vi "RunHTOutconter.vi"() -> ()   [LabVIEW 2012]
uses:
  <vilib>/Utility/file.llb/Read From Spreadsheet File (string).vi
  <vilib>/regexp/Match Regular Expression.xnode
panel:
  out "concatenated string 4":string
  out "filenames":string[](array[string])
  out "concatenated string 3":string
  out "concatenated string 2":string
  out "concatenated string":string
  in  "file path (dialog if empty)":path=path "C:/temp/ht/now/HTentity.txt"
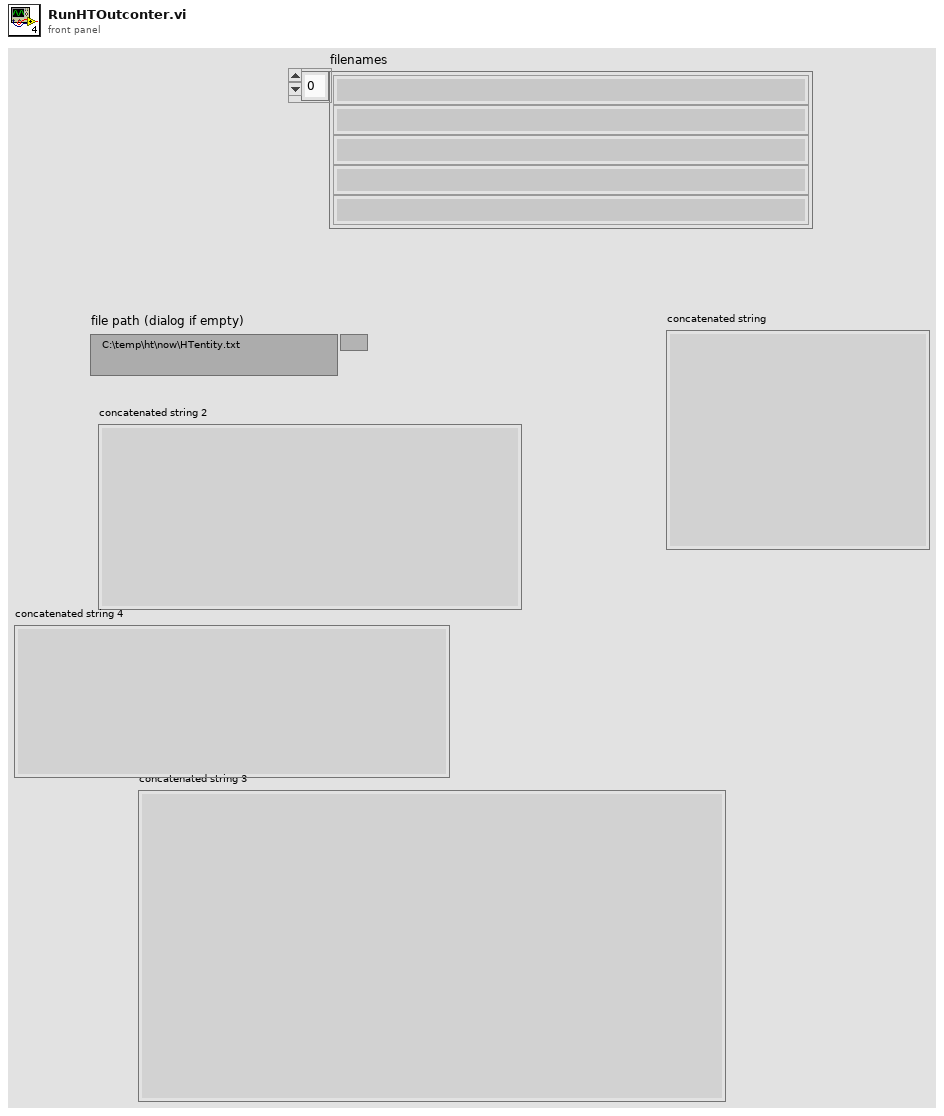
[diagram p1: front panel]
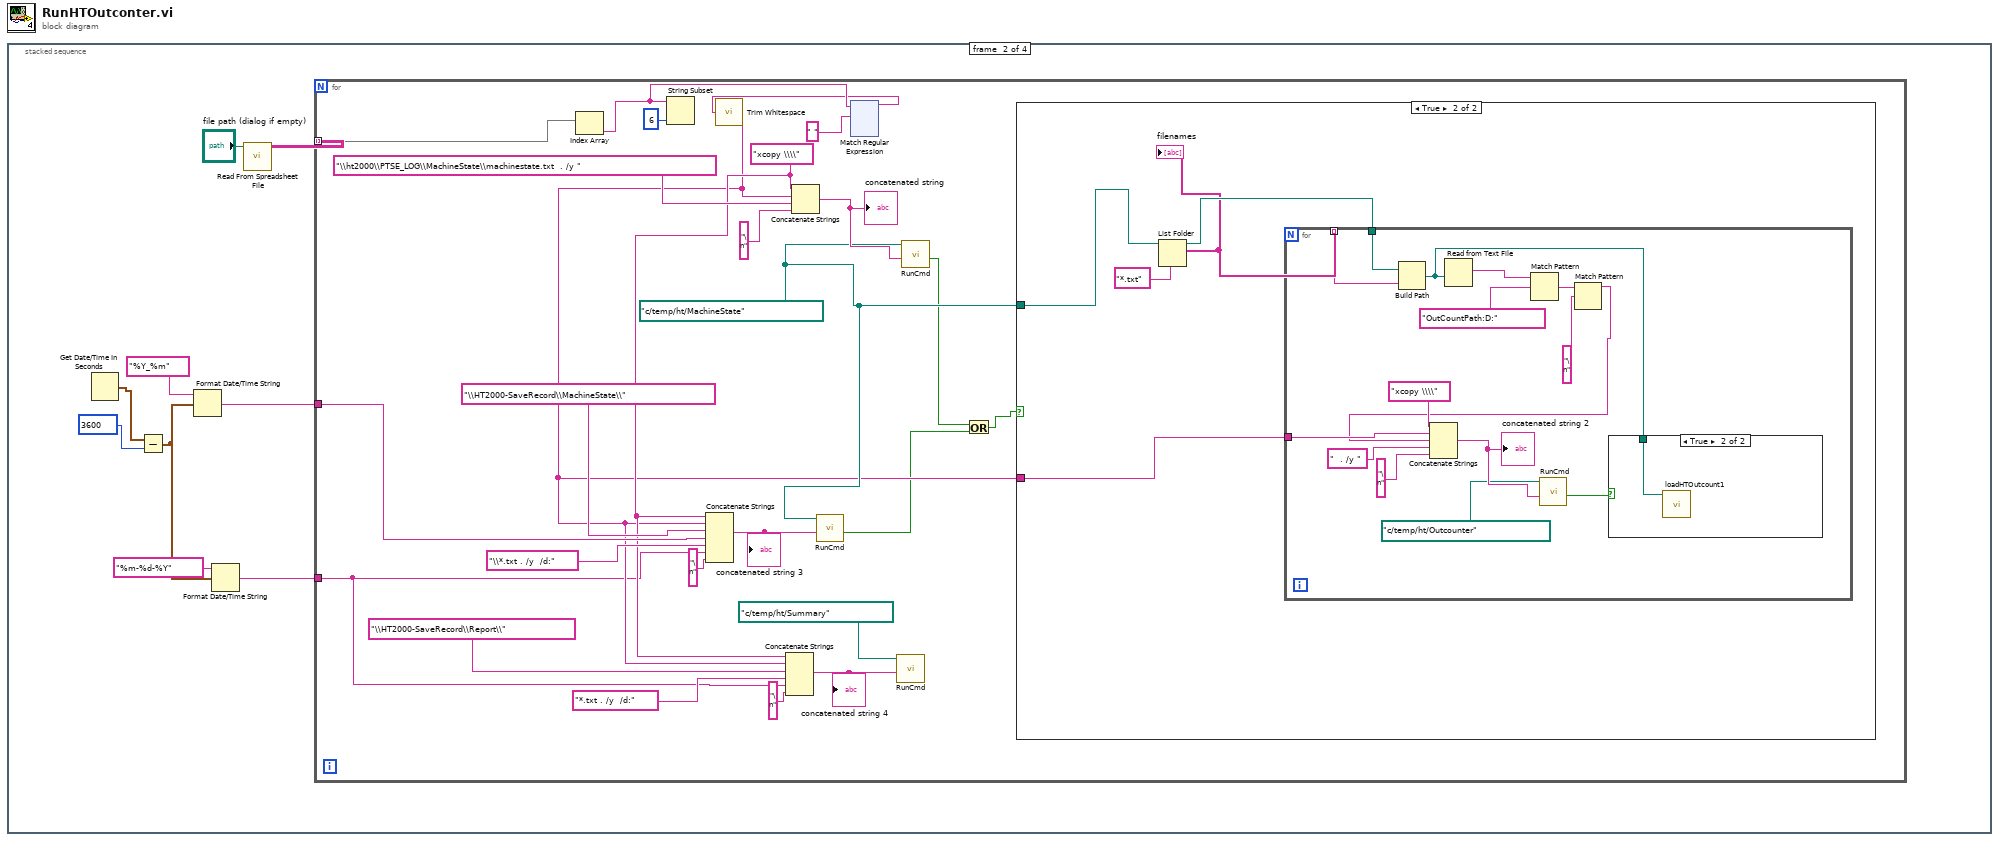
[diagram p0: block diagram]
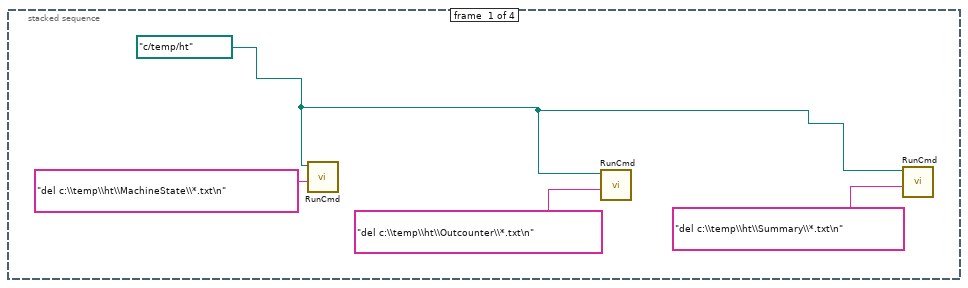
[diagram p2: hidden frame]
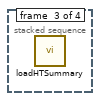
[diagram p5: hidden frame]
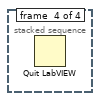
[diagram p6: hidden frame]
diagram:
  n1 = stacked-sequence {
    frame #0 {
      w1 = path "c:/temp/ht" ("working directory")
      n2 = call "RunCmd.vi"("Cmd String"="del c:\\temp\\ht\\MachineState\\*.txt\n", "working directory"=w1) -> ()  [unwired: 8 in, 2 out]
      n3 = call "RunCmd.vi"("Cmd String"="del c:\\temp\\ht\\Outcounter\\*.txt\n", "working directory"=w1) -> ()  [unwired: 8 in, 2 out]
      n4 = call "RunCmd.vi"("Cmd String"="del c:\\temp\\ht\\Summary\\*.txt\n", "working directory"=w1) -> ()  [unwired: 8 in, 2 out]
    }
    frame #1 {
      n5 = Get Date/Time In Seconds() -> (seconds since 1Jan1904=w10:timestamp)
      n6 = Subtract(x=w10, y=3600) -> (x-y=w7:timestamp)
      n7 = Format Date/Time String(time format string (%c)="%Y_%m", seconds (now)=w7) -> (date/time string=w8:string)  [unwired: 1 in]
      n8 = Format Date/Time String(time format string (%c)="%m-%d-%Y", seconds (now)=w7) -> (date/time string=w5:string)  [unwired: 1 in]
      n9 = call-poly <vilib>:"Read From Spreadsheet File.vi"("file path (dialog if empty)"="file path (dialog if empty)") -> ("all rows"=w13:string[][])  [unwired: 6 in, 4 out]
      n10 = for {
        tunnel: w13 -> [w35] mode=indexing
        tunnel: w8 -> [w29]
        tunnel: w5 -> [w19]
        w27 = path "c:/temp/ht/MachineState" ("working directory")
        w23 = "xcopy \\\\" ("string")
        n11 = Index Array(array=w35) -> (element=w33:string)  [unwired: 1 in]
        n12 = String Subset(string=w33, length (rest)=6 ("length (rest)")) -> ()  [unwired: 1 in, 1 out]
        n13 = xnode "Match Regular Expression"("input string"=w33, "regular expression"=" ") -> ("before match"=w32:string)  [unwired: 4 in, 4 out]
        n14 = call <vilib>:"Trim Whitespace.vi"("string"=w32) -> ("trimmed string"=w22:string)  [unwired: 1 in]
        n15 = Concatenate Strings(w23, w22, "\\HT2000-SaveRecord\\MachineState\\" ("string"), w29, "\\*.txt . /y  /d:" ("string"), w19, "\n" ("string")) -> (w26:string)
        "concatenated string 3" <- w26
        n16 = Concatenate Strings(w23, w22, "\\HT2000-SaveRecord\\Report\\" ("string"), "*.txt . /y  /d:" ("string"), w19, "\n" ("string")) -> (w24:string)
        "concatenated string 4" <- w24
        n17 = Concatenate Strings(w23, w22, "\\ht2000\\PTSE_LOG\\MachineState\\machinestate.txt  . /y " ("string"), "\n" ("string")) -> (w37:string)
        "concatenated string" <- w37
        n18 = call "RunCmd.vi"("Cmd String"=w26, "working directory"=w27) -> ("OK"=w14:bool)  [unwired: 8 in, 1 out]
        n19 = call "RunCmd.vi"("Cmd String"=w24, "working directory"=path "c:/temp/ht/Summary") -> ()  [unwired: 8 in, 2 out]
        n20 = call "RunCmd.vi"("Cmd String"=w37, "working directory"=w27) -> ("OK"=w16:bool)  [unwired: 8 in, 1 out]
        n21 = Or(x=w16, y=w14) -> (x .or. y?=w15:bool)
        n22 = case shown="True" w15 {
          tunnel: w27 -> [_ w41]
          tunnel: w22 -> [_ w43]
          frame False {
          }
          frame True {
            n23 = List Folder(path=w41, pattern="*.txt") -> (path out=w40:path, filenames=w39:string[])  [unwired: 2 in, 2 out]
            "filenames" <- w39
            n24 = for {
              tunnel: w43 -> [w54]
              tunnel: w40 -> [w45]
              tunnel: w39 -> [w46] mode=indexing
              n25 = Build Path(base path=w45, name or relative path=w46) -> (appended path=w44:path)
              n26 = Read from Text File(file (use dialog)=w44) -> (text=w53:string)  [unwired: 3 in, 3 out]
              n27 = Match Pattern(string=w53, regular expression="OutCountPath:D:") -> (after substring=w52:string)  [unwired: 1 in, 3 out]
              n28 = Match Pattern(string=w52, regular expression="\n") -> (before substring=w50:string)  [unwired: 1 in, 3 out]
              n29 = Concatenate Strings("xcopy \\\\" ("string"), w54, w50, "  . /y " ("string"), "\n" ("string")) -> (w55:string)
              "concatenated string 2" <- w55
              n30 = call "RunCmd.vi"("Cmd String"=w55, "working directory"=path "c:/temp/ht/Outcounter") -> ("OK"=w48:bool)  [unwired: 8 in, 1 out]
              n31 = case shown="True" w48 {
                tunnel: w44 -> [_ w59]
                frame False {
                }
                frame True {
                  n32 = call "loadHTOutcount1.vi"("file (use dialog)"=w59) -> ()  [unwired: 11 in]
                }
              }
            }
          }
        }
      }
    }
    frame #2 {
      n33 = call "loadHTSummary.vi"() -> ()  [unwired: 12 in]
    }
    frame #3 {
      n34 = Quit LabVIEW() -> ()  [unwired: 1 in]
    }
  }
